vi "Testing 2400.vi"() -> ()   [LabVIEW 2015]
uses:
  <instrlib>/keithley_24xx/Keithley 24XX/Keithley 24XX.lvlib
panel:
  in  "Enable Output (T: Enable)":bool=TRUE
  in  "stop":bool
  in  "Output Level (0)":dbl
  in  "Compliance  Level (0.1)":dbl=0.1
  in  "Source Mode  (0: Voltage)":u16(ring) items=["Voltage", "Current"]
  in  "Output Type  (0: Immediate)":u16(ring) items=["Immediate", "Triggered"]
  in  "VISA resource name":refnum<visa-resource-name>
  out "error out 2400":errorcluster
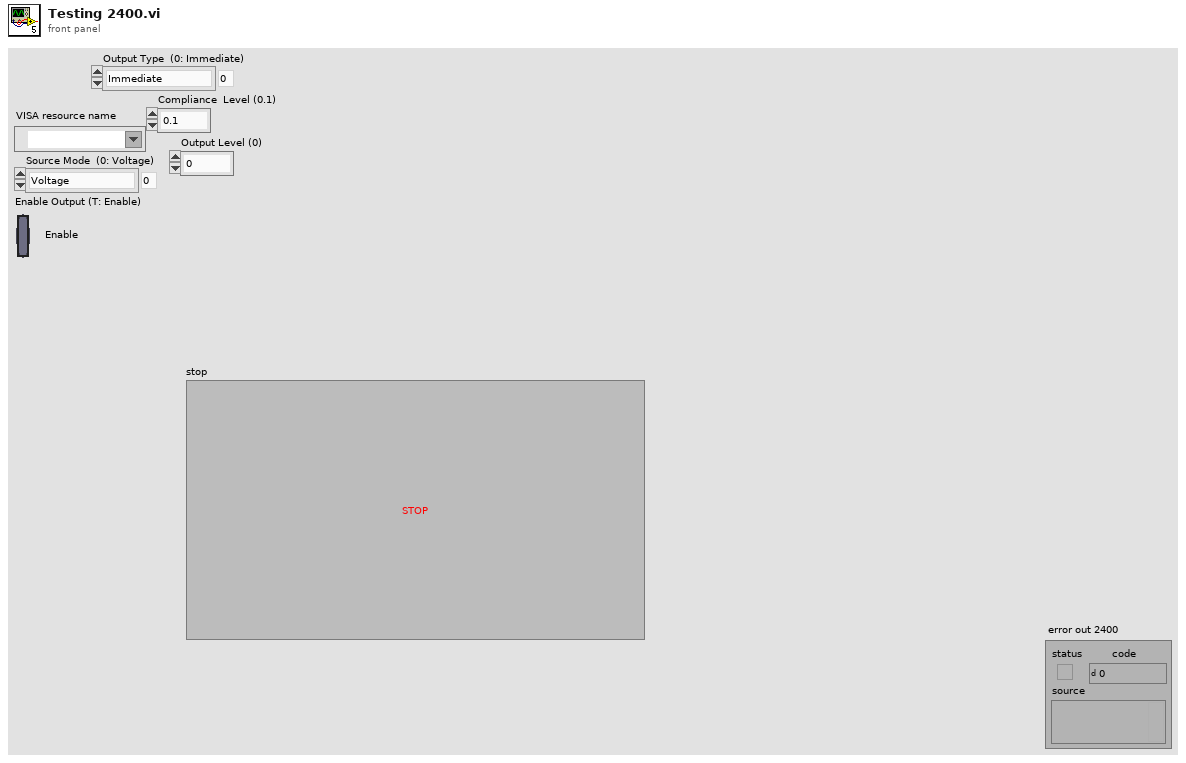
[diagram p1: front panel]
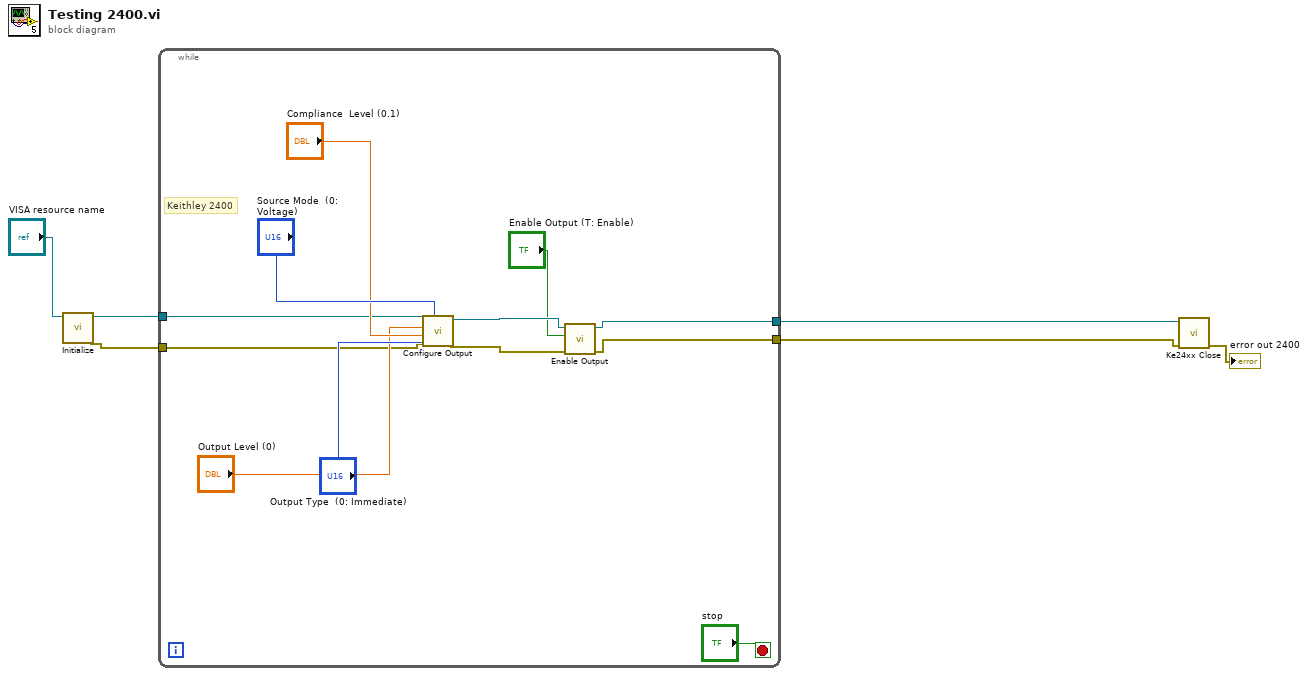
[diagram p0: block diagram]
diagram:
  n1 = call <instrlib>:"Initialize.vi"("VISA resource name"="VISA resource name") -> ("error out"=w1:errorcluster, "VISA resource name out"=w2:refnum<visa-resource-name>)  [unwired: 9 in]
  n2 = while {
    tunnel: [w12] -> w5
    tunnel: [w10] -> w4
    tunnel: w2 -> [w8]
    tunnel: w1 -> [w7]
    stop <- "stop" stop-if-true
    # "Keithley 2400"
    n3 = call <instrlib>:"Configure Output.vi"("Output Type  (0: Immediate)"="Output Type  (0: Immediate)", "Source Mode  (0: Voltage)"="Source Mode  (0: Voltage)", "error in (no error)"=w7, "Compliance  Level (0.1)"="Compliance  Level (0.1)", "Output Level (0)"="Output Level (0)", "VISA resource name"=w8) -> ("error out"=w11:errorcluster, "VISA resource name out"=w13:refnum<visa-resource-name>)  [unwired: 4 in]
    n4 = call <instrlib>:"Enable Output.vi"("error in (no error)"=w11, "Enable Output (T: Enable)"="Enable Output (T: Enable)", "VISA resource name"=w13) -> ("error out"=w10:errorcluster, "VISA resource name out"=w12:refnum<visa-resource-name>)  [unwired: 7 in]
  }
  n5 = call <instrlib>:"Ke24xx Close.vi"("error in (no error)"=w4, "instrument handle"=w5) -> ("error out"=→"error out 2400":errorcluster)  [unwired: 8 in, 1 out]
